vi "Notifier Case Exists.vi"(8 "error in (no error)":errorcluster, 11 "case in":string) -> (0 "error out":errorcluster, 2 "defined case?":bool, 3 "case out":string)   [LabVIEW 2020]
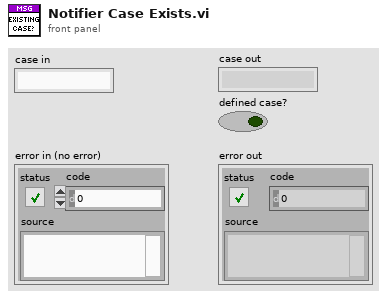
[diagram p1: front panel]
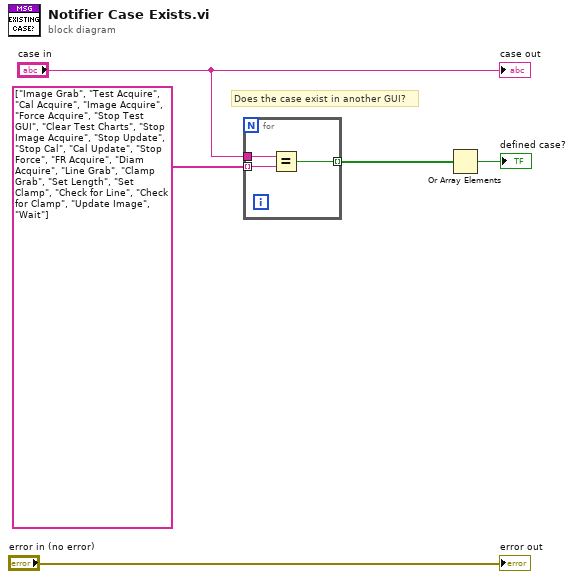
[diagram p0: block diagram]
diagram:
  # "Does the case exist in another GUI?"
  n1 = for {
    tunnel: [w8] -> w3 mode=indexing
    tunnel: "case in" -> [w7]
    tunnel: string[] ["Image Grab", "Test Acquire", "Cal Acquire", "Image Acquire", "Force Acquire", "Stop Test GUI", "Clear Test Charts", "Stop Image Acquire", "Stop Update", "Stop Cal", "Cal Update", "Stop Force", "FR Acquire", "Diam Acquire", "Line Grab", "Clamp Grab", "Set Length", "Set Clamp", "Check for Line", "Check for Clamp", "Update Image", "Wait"] -> [w6] mode=indexing
    n2 = Equal?(x=w7, y=w6) -> (x = y?=w8:bool)
  }
  n3 = Or Array Elements(Boolean array=w3) -> (logical OR=→"defined case?":bool)
  "error out" <- "error in (no error)"
  "case out" <- "case in"
